vi "Configure Output.vi"(8 "error in (no error)":errorcluster, 11 "N5745A in":refnum<class "5745A.lvclass">) -> (0 "error out":errorcluster, 3 "N5745A out":refnum<class "5745A.lvclass">)   [LabVIEW 2018, in "5745A.lvlib" / "5745A.lvclass"]
doc: "This methods is used to turn the N5745A Power Supply ON or OFF."
uses:
  5745A.lvclass
  builds/Power_Supply.lvlibp/Power Supply.lvclass
  C:/Users/Ron.Dexter.LUMINARTECH/Desktop/builds/Power_Supply.lvlibp/Power Supply.lvclass
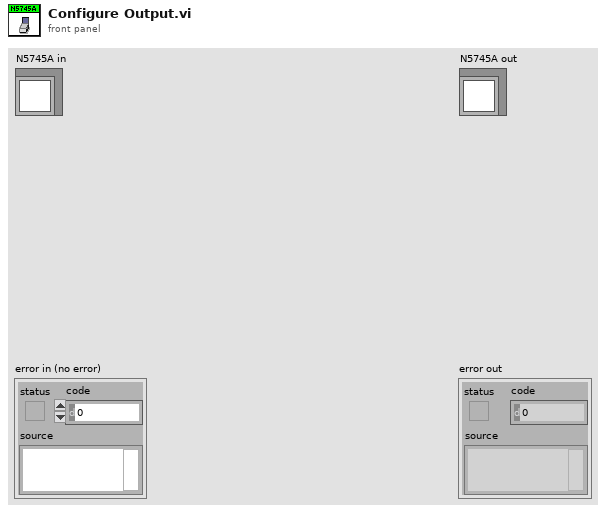
[diagram p1: front panel]
types:
  T1 = typedef "Power_Supply.lvlibp/Supply Settings.ctl" = cluster{"Voltage":dbl, "Current":dbl, "Output":bool}
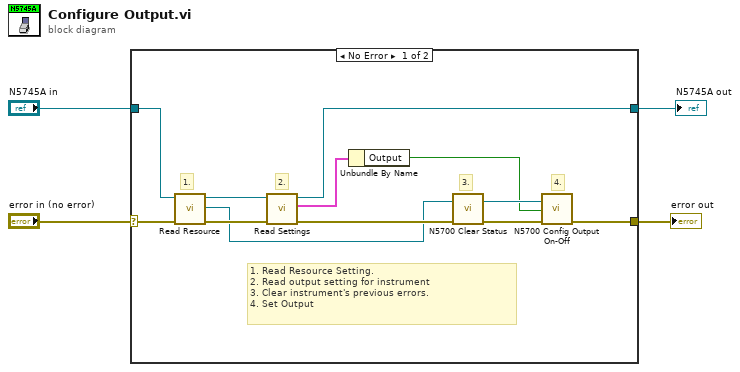
[diagram p0: block diagram]
diagram:
  n1 = case shown="No Error" "error in (no error)" {
    selector: "error in (no error)" -> [w15 w18]
    tunnel: [w12 w18] -> w3
    tunnel: [w10 w17] -> w1
    tunnel: "N5745A in" -> [w16 w17]
    frame No Error {
      # "1. Read Resource Setting.\n2. Read output setting for instrument\n3. Clear instrument's previous errors.\n4. Set Output"
      # "2."
      # "4."
      # "3."
      # "1."
      n2 = call "Read Resource.vi"("error in"=w15, "Power Supply in"=w16) -> ("error out"=w9:errorcluster, "Resource"=w7:refnum<visa-resource-name>, "Power Supply out"=w11:refnum<class "5745A.lvclass">)  [unwired: 7 in]
      n3 = call "Read Settings.vi"("error in (no error)"=w9, "Power Supply in"=w11) -> ("error out"=w8:errorcluster, "Settings"=w6:T1, "Power Supply out"=w10:refnum<class "5745A.lvclass">)  [unwired: 7 in]
      n4 = Unbundle By Name(w6) -> ("Output"=w5:bool)
      n5 = call <instrlib>:"N5700 Clear Status.vi"("error"=w8, "VISA"=w7) -> ("error out"=w14:errorcluster, "VISA out"=w13:refnum<visa-resource-name>)  [unwired: 5 in]
      n6 = call <instrlib>:"N5700 Config Output On-Off.vi"("error"=w14, "Output ON"=w5, "VISA"=w13) -> ("error out"=w12:errorcluster)  [unwired: 4 in, 1 out]
    }
    frame Error {
    }
  }
  "error out" <- w3
  "N5745A out" <- w1
